vi "GObjectDelete.vi"(0 "__args":cluster{"targetVi":string, "uid":i32}) -> (1 "__return":i32, 2 "__errStatus":bool, 3 "__errCode":i32, 4 "__errSource":string)   [LabVIEW 2013]
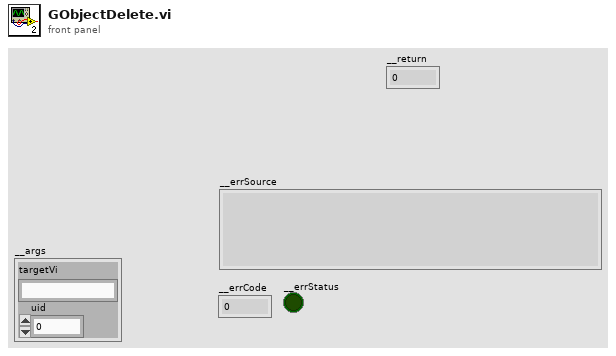
[diagram p1: front panel]
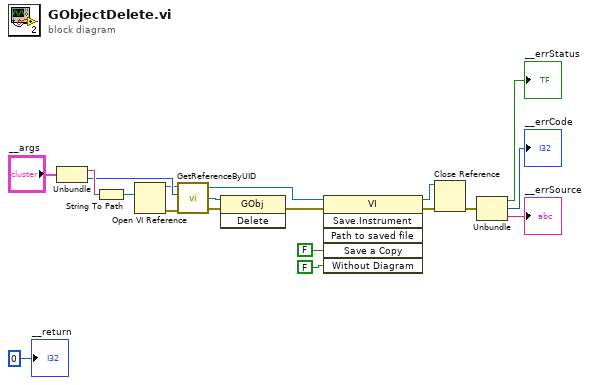
[diagram p0: block diagram]
diagram:
  n1 = Unbundle("__args") -> ("targetVi"=w15:string, "uid"=w12:i32)
  n2 = String To Path(string=w15) -> (path=w14:path)
  n3 = Open VI Reference(vi path=w14) -> (vi reference=w11:refnum<vi>, error out=w1:errorcluster)  [unwired: 5 in]
  n4 = call "GetReferenceByUID.vi"("error in (no error)"=w1, "UID"=w12, "targetVI"=w11) -> ("error out"=w9:errorcluster, "refNum"=w10:refnum<vi>, "dup targetVI"=w7:refnum<vi>)  [unwired: 1 in]
  n5 = invoke class="GObj" method="Delete"(reference=w10, error in=w9) -> (error out=w4:errorcluster)  [unwired: 1 in, 2 out]
  n6 = invoke class="VI" method="Save.Instrument"(reference=w7, error in=w4, "Save a Copy"=FALSE, "Without Diagram"=FALSE) -> (reference out=w8:refnum<vi>, error out=w5:errorcluster)  [unwired: 2 in, 4 out]
  n7 = Close Reference(reference=w8, error in (no error)=w5) -> (error out=w6:errorcluster)
  n8 = Unbundle(w6) -> ("status"=→"__errStatus":bool, "code"=→"__errCode":i32, "source"=→"__errSource":string)
  "__return" <- 0
